vi "Erase Memory.vi"(7 "DUT1?":bool=TRUE, 8 "error in":errorcluster, 9 "Supply PCB over Programator":bool, 10 "Family":string, 11 "6.25":bool) -> (0 "error out":errorcluster, 1 "Erase passed":bool, 2 "standard error":string, 3 "standard output":string)   [LabVIEW 2023]
panel:
  out "return code":i32
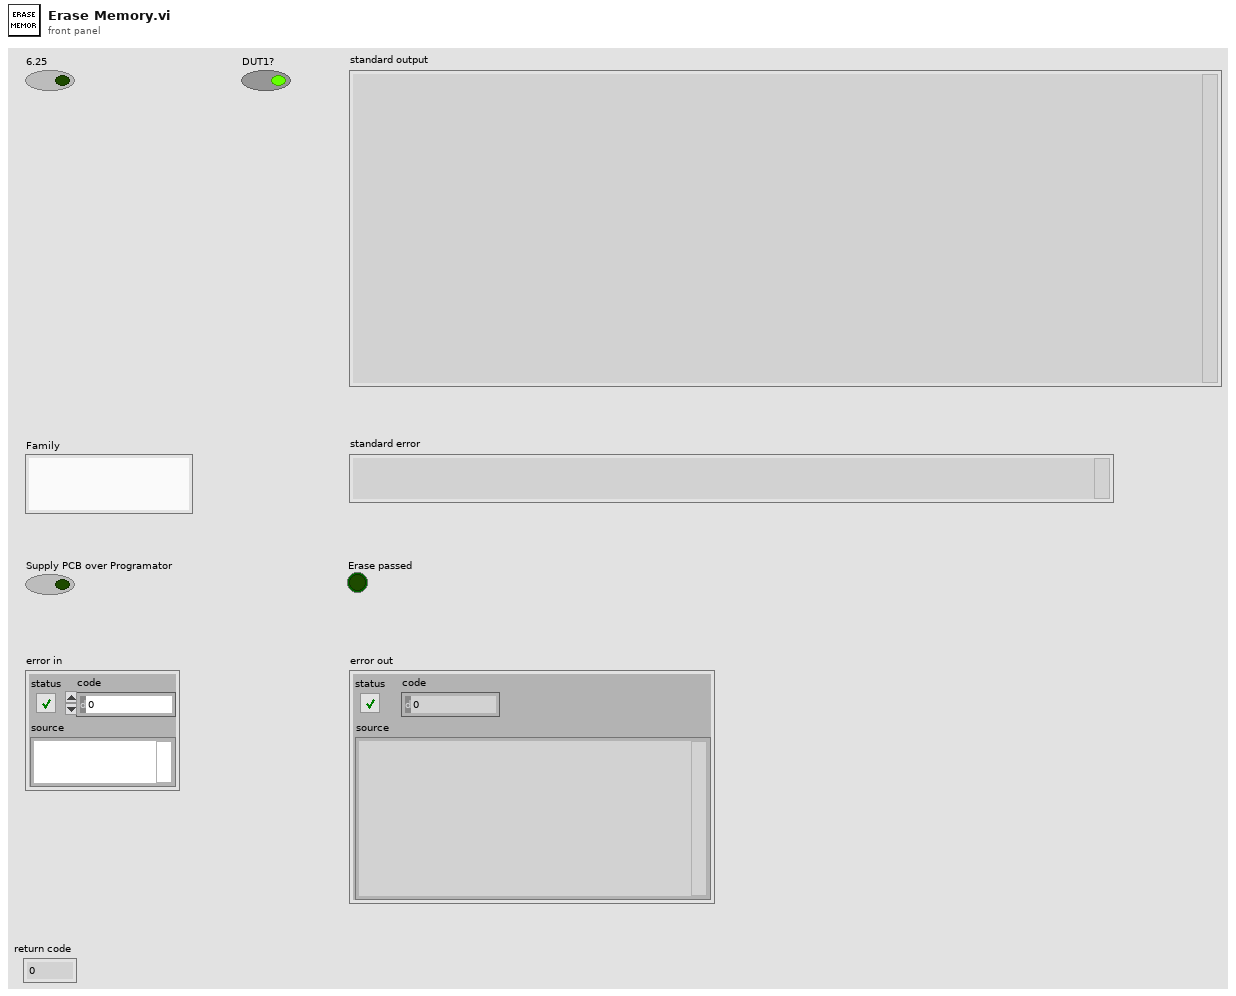
[diagram p1: front panel]
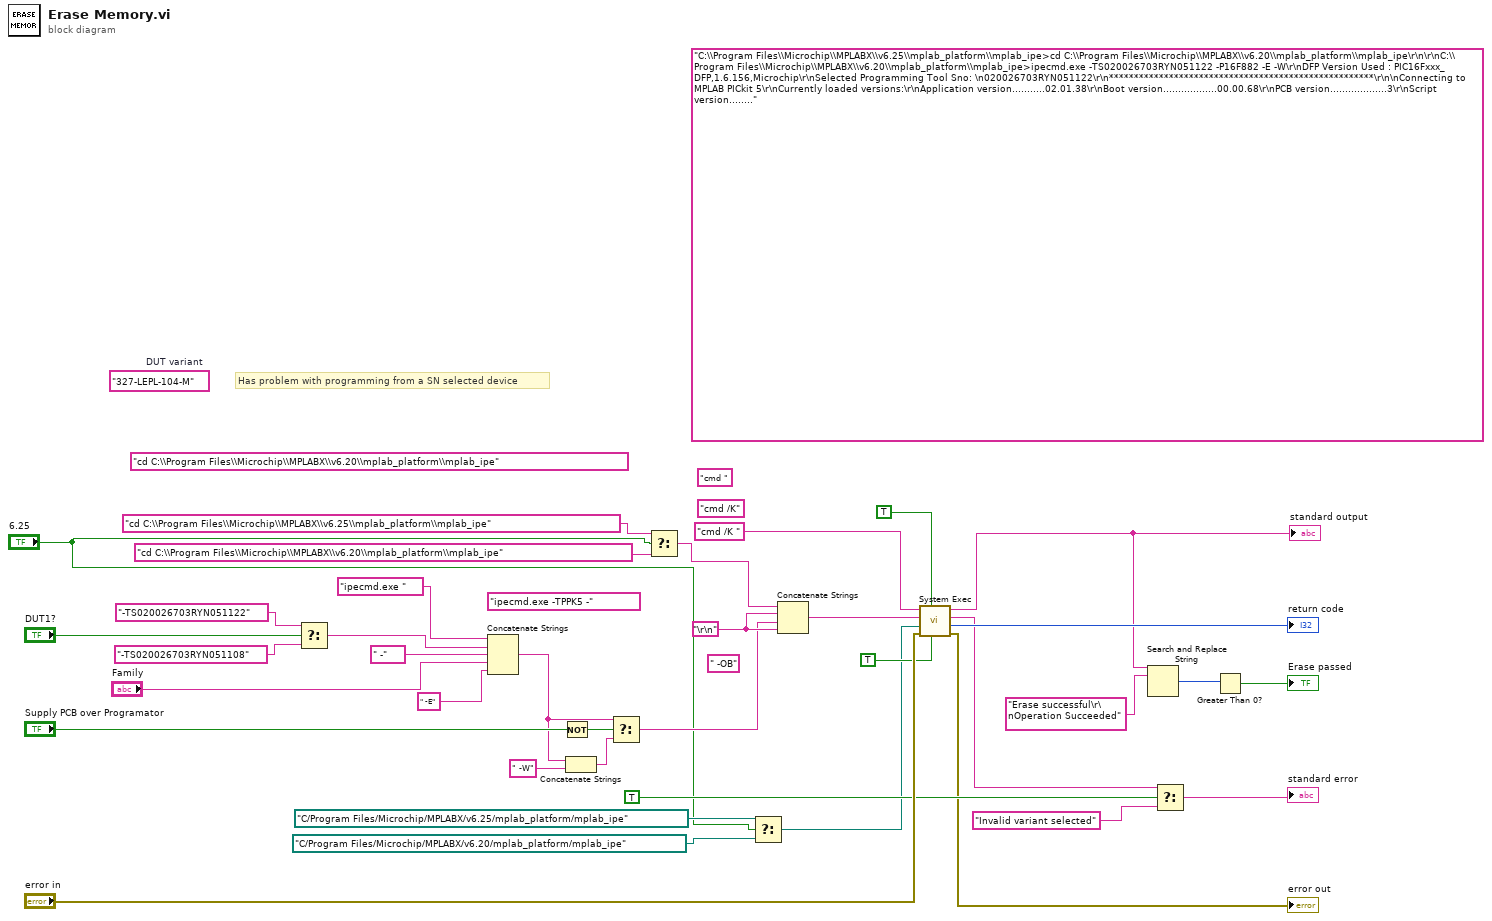
[diagram p0: block diagram]
diagram:
  (unwired) "cd C:\\Program Files\\Microchip\\MPLABX\\v6.20\\mplab_platform\\mplab_ipe" ("command line")
  (unwired) "C:\\Program Files\\Microchip\\MPLABX\\v6.25\\mplab_platform\\mplab_ipe>cd C:\\Program Files\\Microchip\\MPLABX\\v6.20\\mplab_platform\\mplab_ipe\r\n\r\nC:\\Program Files\\Microchip\\MPLABX\\v6.20\\mplab_platform\\mplab_ipe>ipecmd.exe -TS020026703RYN051122 -P16F882 -E -W\r\nDFP Version Used : PIC16Fxxx_DFP,1.6.156,Microchip\r\nSelected Programming Tool Sno: \n020026703RYN051122\r\n*****************************************************\r\n\nConnecting to MPLAB PICkit 5\r\nCurrently loaded versions:\r\nApplication version...........02.01.38\r\nBoot version..................00.00.68\r\nPCB version...................3\r\nScript version................00.06.71\r\nScript build number...........74cdf38a4d\r\nTool pack version ............2.3.327\r\nPICkit 5 is supplying power to the target (5.00 volts).\r\nTarget device PIC16F882 found.\r\nDevice Revision Id  = 0x0\r\nDevice Id = 0x2000\r\n*****************************************************\r\nErasing...\r\nErase successful\r\nOperation Succeeded\r\n\r\nC:\\Program Files\\Microchip\\MPLABX\\v6.20\\mplab_platform\\mplab_ipe>" ("standard output 2")
  (unwired) "cmd " ("command line")
  (unwired) "ipecmd.exe -TPPK5 -" ("command line")
  (unwired) "cmd /K" ("command line")
  (unwired) " -OB" ("string")
  (unwired) "327-LEPL-104-M"  # DUT variant
  w22 = "\r\n"
  # "Has problem with programming from a SN selected device"
  n1 = Select(t="-TS020026703RYN051122" ("command line"), s="DUT1?", f="-TS020026703RYN051108" ("command line")) -> (s? t:f=w11:string)
  n2 = Concatenate Strings("ipecmd.exe " ("command line"), w11, " -" ("command line"), "Family", " -E" ("string")) -> (w17:string)
  n3 = Not(x="Supply PCB over Programator") -> (.not. x?=w32:bool)
  n4 = Concatenate Strings(w17, " -W" ("string")) -> (w19:string)
  n5 = Select(t=w17, s=w32, f=w19) -> (s? t:f=w21:string)
  n6 = Select(t="cd C:\\Program Files\\Microchip\\MPLABX\\v6.25\\mplab_platform\\mplab_ipe" ("command line"), s="6.25", f="cd C:\\Program Files\\Microchip\\MPLABX\\v6.20\\mplab_platform\\mplab_ipe" ("command line")) -> (s? t:f=w1:string)
  n7 = Select(t=path "C:/Program Files/Microchip/MPLABX/v6.25/mplab_platform/mplab_ipe" ("working directory"), s="6.25", f=path "C:/Program Files/Microchip/MPLABX/v6.20/mplab_platform/mplab_ipe" ("working directory")) -> (s? t:f=w2:path)
  n8 = Concatenate Strings(w1, w22, w21, w22) -> (w35:string)
  n9 = call <vilib>:"System Exec.vi"("run minimized? (F)"=TRUE, "wait until completion? (T)"=TRUE, "error in (no error)"="error in", "working directory"=w2, "standard input"=w35, "command line"="cmd /K ") -> ("error out"=→"error out":errorcluster, "return code"=→"return code":i32, "standard error"=w28:string, "standard output"=w26:string)  [unwired: 2 in]
  "standard output" <- w26
  n10 = Search and Replace String(input string=w26, search string="Erase successful\r\nOperation Succeeded" ("standard output 2")) -> (number of replacements=w25:i32)  [unwired: 6 in, 3 out]
  n11 = Select(t=w28, s=TRUE, f="Invalid variant selected") -> (s? t:f=→"standard error":string)
  n12 = Greater Than 0?(x=w25) -> (x > 0?=→"Erase passed":bool)
